vi "TEST_Color.vi"() -> ()   [LabVIEW 2021, in "Picture2D.lvlib"]
uses:
  Picture2D/Picture2D.lvlib
  ColorRGB/ColorRGB.lvclass
  ColorHSL/ColorHSL.lvclass
  ColorCMYK/ColorCMYK.lvclass
  ColorHSV/ColorHSV.lvclass
  ColorGrayScale/ColorGrayScale.lvclass
panel:
  out "Gray Scale":u32(colorbox)
  out "HSV Color Match":bool
  out "H (°)":dbl format="%#_3p"
  out "HSV Color":u32(colorbox)
  out "HSV error out":errorcluster
  out "V (%)":dbl format="%#_3p"
  out "S (%)":dbl format="%#_3p"
  out "CMYK Color Match":bool
  out "RGB Color Match":bool
  out "HSL Color Match":bool
  out "CMYK Color":u32(colorbox)
  out "error out":errorcluster
  out "K (%)":dbl
  out "Y (%)":dbl
  out "M (%)":dbl
  out "C (%)":dbl
  out "H (°)":dbl format="%#_3p"
  out "B":u8
  out "G":u8
  out "R":u8
  out "HSL Color":u32(colorbox)
  out "HSL error out":errorcluster
  out "L (%)":dbl format="%#_3p"
  out "S (%)":dbl format="%#_3p"
  out "RGB Color":u32(colorbox)
  out "RGB error out":errorcluster
  in  "Color":u32(colorbox)
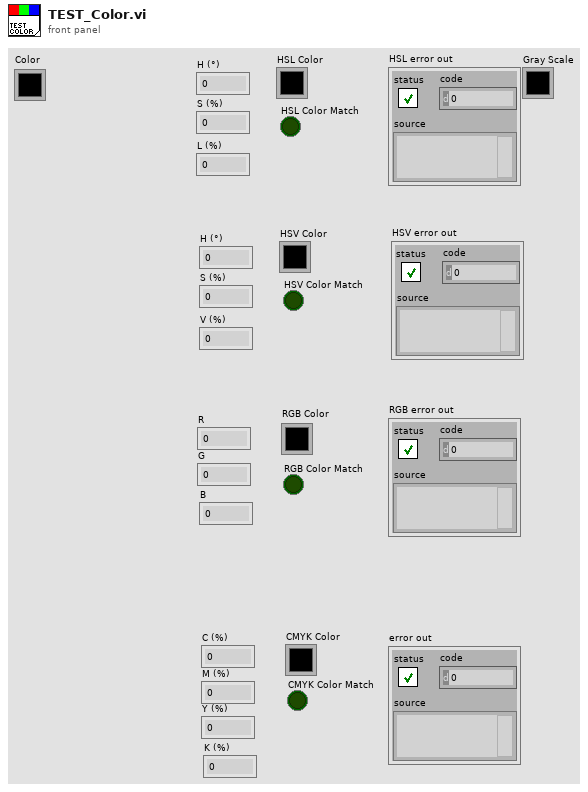
[diagram p1: front panel]
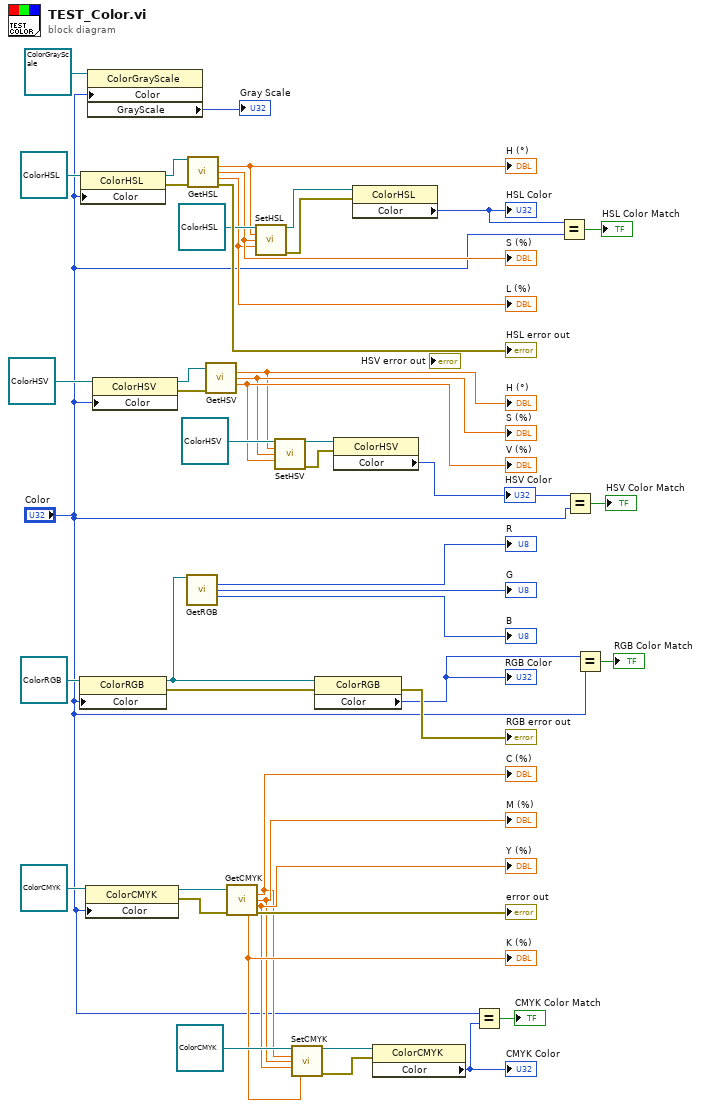
[diagram p0: block diagram]
diagram:
  n1 = property class="ColorRGB"(reference=refnum<class "ColorRGB.lvclass"> refnum ("ColorRGB in"), "Color"="Color") -> (reference out=w37:refnum<class "ColorRGB.lvclass">, error out=w22:errorcluster)  [unwired: 1 in]
  n2 = property class="ColorHSL"(reference=refnum<class "ColorHSL.lvclass"> refnum ("Picture2D.lvlib:ColorHSL"), "Color"="Color") -> (reference out=w46:refnum<class "ColorHSL.lvclass">, error out=w44:errorcluster)  [unwired: 1 in]
  n3 = property class="ColorCMYK"(reference=refnum<class "ColorCMYK.lvclass"> refnum ("Picture2D.lvlib:ColorRGB"), "Color"="Color") -> (reference out=w32:refnum<class "ColorCMYK.lvclass">, error out=w31:errorcluster)  [unwired: 1 in]
  n4 = property class="ColorGrayScale"(reference=refnum<class "ColorGrayScale.lvclass"> refnum ("Picture2D.lvlib:ColorGrayScale"), "Color"="Color") -> ("GrayScale"=→"Gray Scale":u32)  [unwired: 1 in, 2 out]
  n5 = property class="ColorHSV"(reference=refnum<class "ColorHSV.lvclass"> refnum ("Picture2D.lvlib:ColorHSV"), "Color"="Color") -> (reference out=w12:refnum<class "ColorHSV.lvclass">, error out=w11:errorcluster)  [unwired: 1 in]
  n6 = call-dynamic "GetRGB.vi"("ColorRGB in"=w37) -> ("R"=→"R":u8, "G"=→"G":u8, "B"=→"B":u8)  [unwired: 10 in, 2 out]
  n7 = call-dynamic "GetHSL.vi"("ColorHLS in"=w46, "error in (no error)"=w44) -> ("H (°)"=w42:dbl, "S (%)"=w41:dbl, "L (%)"=w40:dbl, "error out"=→"HSL error out":errorcluster)  [unwired: 9 in, 1 out]
  "S (%)" <- w41
  "L (%)" <- w40
  "H (°)" <- w42
  n8 = call-dynamic "GetHSV.vi"("ColorHLV in"=w12, "error in (no error)"=w11) -> ("H (°)"=w7:dbl, "S (%)"=w8:dbl, "V (%)"=w9:dbl)  [unwired: 9 in, 2 out]
  "S (%)" <- w8
  "V (%)" <- w9
  "H (°)" <- w7
  n9 = call-dynamic "GetCMYK.vi"("ColorCMYK in"=w32, "error in (no error)"=w31) -> ("C (%)"=w24:dbl, "M (%)"=w25:dbl, "Y (%)"=w26:dbl, "K (%)"=w27:dbl, "error out"=→"error out":errorcluster)  [unwired: 8 in, 1 out]
  "C (%)" <- w24
  "M (%)" <- w25
  "Y (%)" <- w26
  "K (%)" <- w27
  n10 = call-dynamic "SetHSL.vi"("ColorHLS in"=refnum<class "ColorHSL.lvclass"> refnum ("Picture2D.lvlib:ColorHSL"), "H"=w42, "S"=w41, "L"=w40) -> ("ColorHLS out"=w39:refnum<class "ColorHSL.lvclass">, "error out"=w38:errorcluster)  [unwired: 10 in]
  n11 = call-dynamic "SetHSV.vi"("ColorHLS in"=refnum<class "ColorHSV.lvclass"> refnum ("Picture2D.lvlib:ColorHSV"), "H"=w7, "S"=w8, "V"=w9) -> ("ColorHLS out"=w6:refnum<class "ColorHSV.lvclass">, "error out"=w5:errorcluster)  [unwired: 10 in]
  n12 = call-dynamic "SetCMYK.vi"("ColorRGB in"=refnum<class "ColorCMYK.lvclass"> refnum ("Picture2D.lvlib:ColorRGB"), "C (%)"=w24, "M (%)"=w25, "Y (%)"=w26, "K (%)"=w27) -> ("ColorRGB out"=w28:refnum<class "ColorCMYK.lvclass">, "error out"=w23:errorcluster)  [unwired: 9 in]
  n13 = property class="ColorRGB"(reference=w37, error in=w22) -> (error out=→"RGB error out":errorcluster, "Color"=w16:u32)  [unwired: 1 out]
  "RGB Color" <- w16
  n14 = property class="ColorHSV"(reference=w6, error in=w5) -> ("Color"=w4:u32)  [unwired: 2 out]
  "HSV Color" <- w4
  n15 = property class="ColorHSL"(reference=w39, error in=w38) -> ("Color"=w20:u32)  [unwired: 2 out]
  "HSL Color" <- w20
  n16 = property class="ColorCMYK"(reference=w28, error in=w23) -> ("Color"=w18:u32)  [unwired: 2 out]
  "CMYK Color" <- w18
  n17 = Equal?(x="Color", y=w18) -> (x = y?=→"CMYK Color Match":bool)
  n18 = Equal?(x=w20, y="Color") -> (x = y?=→"HSL Color Match":bool)
  n19 = Equal?(x=w4, y="Color") -> (x = y?=→"HSV Color Match":bool)
  n20 = Equal?(x=w16, y="Color") -> (x = y?=→"RGB Color Match":bool)
